vi "Test_API_InitDone_NoError.vi"(8 "error in (no error)":errorcluster, 11 "TestCase in":refnum<class "TestComposedLog.lvclass">) -> (0 "error out":errorcluster, 3 "TestCase out":refnum<class "TestComposedLog.lvclass">)   [LabVIEW 2017, in "TestComposedLog.lvclass"]
uses:
  TestComposedLog.lvclass
  Source/Composed Log/LoggerReference/LoggerReference.lvclass/LoggerReference.ctl
  f210135d-4f31-415a-94e1-f6ce2d6b5d86.vi
  f210135d-4f31-415a-94e1-f6ce2d6b5d86.vi/0729fb90-d539-444e-88b3-5ec12ff95ee5.vi
  Source/Composed Log/LoggerReference/Return Aggregate Queues.vi
  Source/Composed Log/LoggerReference/Add Aggregate Log.vi
  f210135d-4f31-415a-94e1-f6ce2d6b5d86.vi/0729fb90-d539-444e-88b3-5ec12ff95ee5.vi/9d2819f5-b4ce-4e7b-bc5c-22c38081e13b.vi
  Source/Composed Log/LoggerReference/Send Add Sink.vi
  Source/LVQueue Sink/LVQueue Sink.lvclass
  C:/CS/Internal/LabVIEW/Logger/Source/Composed Log/Log Sink/Log Sink.lvclass
  Source/Composed Log/Application Logger/Launch Worker Loop.vi
  Source/Composed Log/LoggerReference/Initialize Logger Instance.vi
  Source/Composed Log/Singleton Event Log/Logger Queue FGV.vi
  Source/Composed Log/IErrorFormat/IErrorFormat.lvclass
  Source/Composed Log/LoggerReference/LoggerReference.lvclass
  Source/Composed Log/Log Sink/Log Sink.lvclass
  <vilib>/addons/_JKI Toolkits/VI Tester/TestCase.llb/TestCase.lvclass
  Source/Composed Log/Singleton Event Log/Singleton Event Log.lvlib
  C:/Program Files (x86)/National Instruments/LabVIEW 2017/vi.lib/addons/_JKI Toolkits/VI Tester/TestCase.llb/TestCase.lvclass
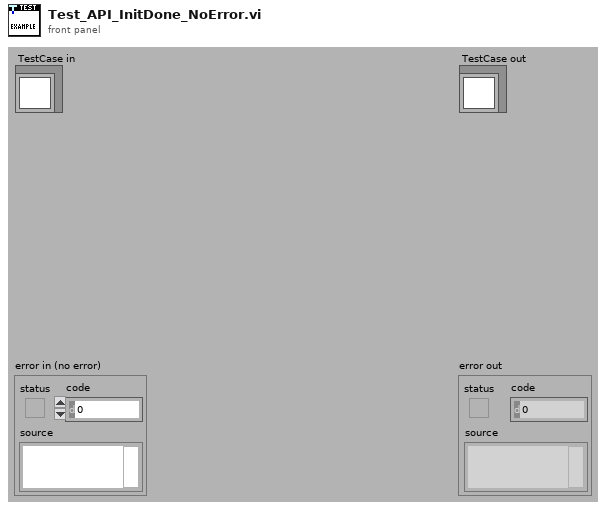
[diagram p1: front panel]
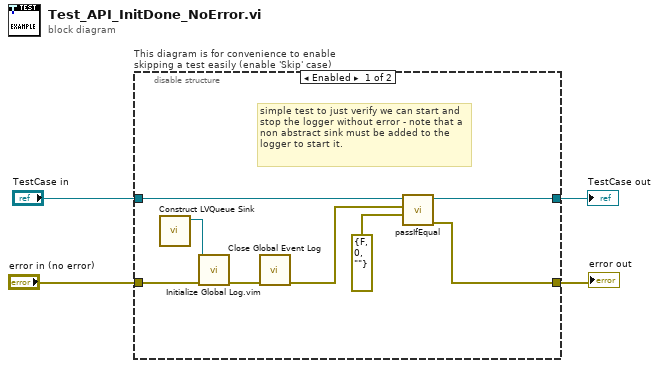
[diagram p0: block diagram]
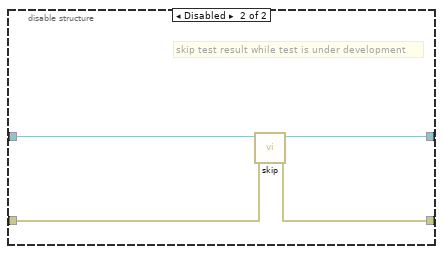
[diagram p2: hidden frame]
diagram:
  n1 = disable-structure "This diagram is for convenience to enable skipping a test easily (enable 'Skip' case)" shown="Enabled" {
    disable-tunnel: "TestCase in" -> [w10 w16]
    disable-tunnel: [w11 w14] -> w1
    disable-tunnel: [w7 w15] -> w3
    disable-tunnel: "error in (no error)" -> [w6 w13]
    frame Enabled {
      # "simple test to just verify we can start and stop the logger without error - note that a non abstract sink must be added to the logger to start it."
      n2 = call "Construct LVQueue Sink.vi"() -> ("LVQueue Sink out"=w5:refnum<class "LVQueue Sink.lvclass">)  [unwired: 10 in, 1 out]
      n3 = call "Initialize Global Log.vim"("error in (no error)"=w6, "Log Sink(s)"=w5) -> ("error out"=w12:errorcluster)  [unwired: 8 in, 1 out]
      n4 = call "Close Global Event Log.vi"("error in (no error)"=w12) -> ("error out"=w8:errorcluster)  [unwired: 10 in]
      n5 = call-dynamic "passIfEqual.vi"("y"=errorcluster {"status"=FALSE, "code"=0, "source"=""} ("error out"), "x"=w8, "TestCase in"=w10) -> ("error out"=w7:errorcluster, "TestCase out"=w11:refnum<class "TestComposedLog.lvclass">)  [unwired: 7 in]
    }
    frame Disabled {
      # "skip test result while test is under development"
      n6 = call <vilib>:"skip.vi"("error in (no error)"=w13, "TestCase in"=w16) -> ("error out"=w15:errorcluster, "TestCase out"=w14:refnum<class "TestComposedLog.lvclass">)  [unwired: 8 in]
    }
  }
  "error out" <- w3
  "TestCase out" <- w1
